vi "N5232-ReadAverageMode.vi"(0 "Session In":refnum<visa-resource-name>="TCPIP0::169.254.70.180::inst0::INSTR", 11 "error in":errorcluster {"code" format="%.0x"}, 13 "Chan":i32=1) -> (4 "Session Out":refnum<visa-resource-name>, 6 "AvgCount?":string, 8 "AvgState?":string, 10 "AvgMode?":string, 15 "error out":errorcluster {"code" format="%.0x"})   [LabVIEW 2018]
doc: "Launches the Instrument I/O Assistant, which you can use to communicate with message-based instruments and graphically parse the response. For example you can communicate with an instrument that uses a serial, Ethernet, or GPIB interface."
uses:
  Keysight PNA Series/Keysight PNA Series.lvlib
panel:
  out "Error Message":string
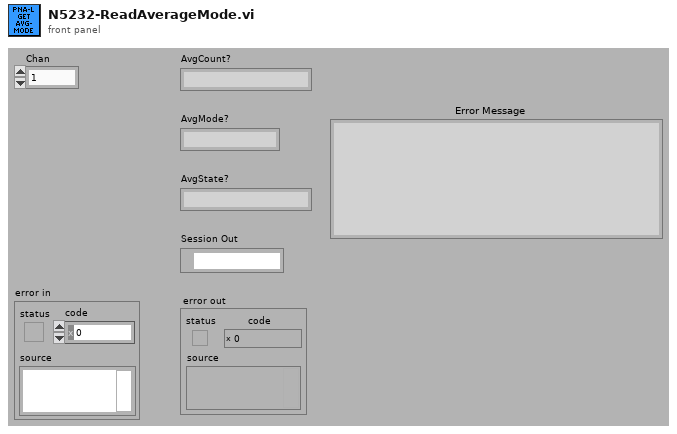
[diagram p1: front panel]
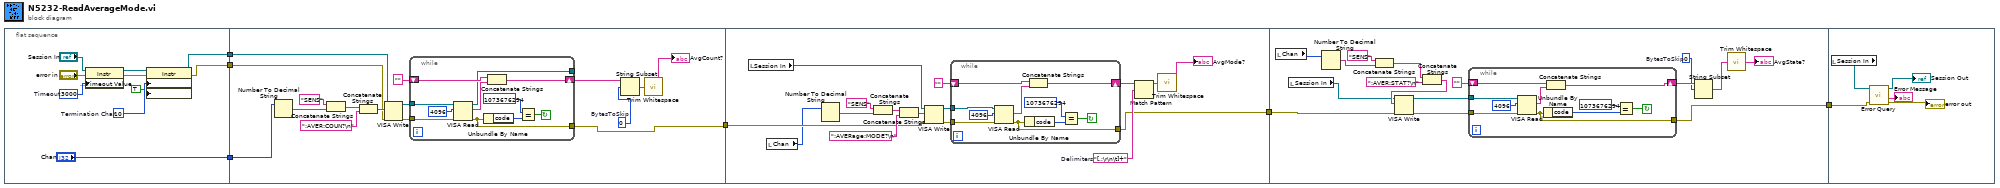
[diagram p0: block diagram]
diagram:
  n1 = flat-sequence {
    tunnel: [w8] -> w4
    tunnel: [w9] -> w3
    tunnel: ["Chan"] -> w2
    tunnel: [w19] -> w5
    tunnel: w4 -> [w22]
    tunnel: w3 -> [w21]
    tunnel: w2 -> [w18]
    tunnel: [w47] -> w6
    tunnel: w5 -> [w49]
    tunnel: w6 -> [w85]
    tunnel: [w71] -> w1
    tunnel: w1 -> [w100]
    frame #0 {
      w12 = u8 10  # Termination Char
      w10 = u32 3000  # Timeout
      n2 = property class="Instr"(reference="Session In", error in="error in", "General Settings:Timeout Value"=w10) -> (reference out=w16:refnum<visa-resource-name>, error out=w15:errorcluster)
      n3 = property class="Instr"(reference=w16, error in=w15, "Message Based Settings:Termination Character"=w12, "Message Based Settings:Termination Character Enable"=TRUE ("enable")) -> (reference out=w9:refnum<visa-resource-name>, error out=w8:errorcluster)
    }
    frame #1 {
      w25 = 0  # BytesToSkip
      n4 = Number To Decimal String(number=w18) -> (decimal integer string=w26:string)  [unwired: 1 out]
      n5 = Concatenate Strings("SENS" ("staticText"), w26) -> (w29:string)
      n6 = Concatenate Strings(w29, ":AVER:COUN?\n" ("StaticText")) -> (w28:string)
      n7 = VISA Write(VISA resource name=w21, write buffer=w28, error in (no error)=w22) -> (VISA resource name out=w32:refnum<visa-resource-name>, error out=w27:errorcluster)  [unwired: 1 out]
      n8 = while {
        tunnel: w32 -> [w34]
        shift-left: "" -> [w37]
        shift-right: [w36] -> w31
        tunnel: w27 -> [w35]
        tunnel: [w39] -> w19
        tunnel: [w33] -> _
        stop <- w41 continue-if-true
        n9 = VISA Read(VISA resource name=w34, byte count=u32 4096 ("byte count (0)"), error in (no error)=w35) -> (VISA resource name out=w33:refnum<visa-resource-name>, read buffer=w38:string, error out=w39:errorcluster)  [unwired: 1 out]
        n10 = Unbundle By Name(w39) -> ("code"=w42:i32)
        n11 = Concatenate Strings(w37, w38) -> (w36:string)
        n12 = Equal?(x=1073676294, y=w42) -> (x = y?=w41:bool)
      }
      n13 = String Subset(string=w31, offset (0)=w25) -> (substring=w30:string)  [unwired: 1 out]
      n14 = call <vilib>:"Trim Whitespace.vi"("string"=w30) -> ("trimmed string"=→"AvgCount?":string)  [unwired: 1 in]
    }
    frame #2 {
      w52 = "[,;\r\n\t]+"  # Delimiters
      n15 = local read "Session In"() -> (w46:refnum<visa-resource-name>)
      n16 = local read "Chan"() -> (w45:i32)
      n17 = Number To Decimal String(number=w45) -> (decimal integer string=w53:string)  [unwired: 1 out]
      n18 = Concatenate Strings("SENS" ("staticText"), w53) -> (w56:string)
      n19 = Concatenate Strings(w56, ":AVERage:MODE?\n" ("StaticText")) -> (w55:string)
      n20 = VISA Write(VISA resource name=w46, write buffer=w55, error in (no error)=w49) -> (VISA resource name out=w59:refnum<visa-resource-name>, error out=w54:errorcluster)  [unwired: 1 out]
      n21 = while {
        tunnel: w59 -> [w60]
        shift-left: "" -> [w63]
        shift-right: [w62] -> w58
        tunnel: w54 -> [w61]
        tunnel: [w65] -> w47
        stop <- w67 continue-if-true
        n22 = VISA Read(VISA resource name=w60, byte count=u32 4096 ("byte count (0)"), error in (no error)=w61) -> (read buffer=w64:string, error out=w65:errorcluster)  [unwired: 2 out]
        n23 = Unbundle By Name(w65) -> ("code"=w68:i32)
        n24 = Concatenate Strings(w63, w64) -> (w62:string)
        n25 = Equal?(x=1073676294, y=w68) -> (x = y?=w67:bool)
      }
      n26 = Match Pattern(string=w58, regular expression=w52) -> (before substring=w57:string)  [unwired: 4 out]
      n27 = call <vilib>:"Trim Whitespace.vi"("string"=w57) -> ("trimmed string"=→"AvgMode?":string)  [unwired: 1 in]
    }
    frame #3 {
      w75 = 0  # BytesToSkip
      n28 = local read "Chan"() -> (w72:i32)
      n29 = local read "Session In"() -> (w73:refnum<visa-resource-name>)
      n30 = Number To Decimal String(number=w72) -> (decimal integer string=w84:string)  [unwired: 1 out]
      n31 = Concatenate Strings("SENS" ("staticText"), w84) -> (w80:string)
      n32 = Concatenate Strings(w80, ":AVER:STAT?\n" ("StaticText")) -> (w81:string)
      n33 = VISA Write(VISA resource name=w73, write buffer=w81, error in (no error)=w85) -> (VISA resource name out=w74:refnum<visa-resource-name>, error out=w82:errorcluster)  [unwired: 1 out]
      n34 = while {
        tunnel: w74 -> [w86]
        shift-left: "" -> [w89]
        shift-right: [w88] -> w76
        tunnel: w82 -> [w87]
        tunnel: [w91] -> w71
        stop <- w93 continue-if-true
        n35 = VISA Read(VISA resource name=w86, byte count=u32 4096 ("byte count (0)"), error in (no error)=w87) -> (read buffer=w90:string, error out=w91:errorcluster)  [unwired: 2 out]
        n36 = Unbundle By Name(w91) -> ("code"=w94:i32)
        n37 = Concatenate Strings(w89, w90) -> (w88:string)
        n38 = Equal?(x=1073676294, y=w94) -> (x = y?=w93:bool)
      }
      n39 = String Subset(string=w76, offset (0)=w75) -> (substring=w77:string)  [unwired: 1 out]
      n40 = call <vilib>:"Trim Whitespace.vi"("string"=w77) -> ("trimmed string"=→"AvgState?":string)  [unwired: 1 in]
    }
    frame #4 {
      n41 = local read "Session In"() -> (w96:refnum<visa-resource-name>)
      n42 = call "Error Query.vi"("error in (no error)"=w100, "VISA resource name"=w96) -> ("error out"=→"error out":errorcluster, "Error Message"=→"Error Message":string, "VISA resource name out"=→"Session Out":refnum<visa-resource-name>)  [unwired: 6 in, 1 out]
    }
  }
